vi "Servo Log change.vi"(10 "Servo variables Now":T3, 11 "Servo variables Before":T3) -> (2 "Changes":T1[](array[typedef]), 3 "Any change?":bool)   [LabVIEW 2017, in "Servo drive module.lvlib"]
doc: "Compares previous and current status variables of servo drives. Changes are concated into and array.\nparams:\nServo variables before\nServo variables now\nreturs:\nChanges"
uses:
  Servo drive module.lvlib
  ctl/Servo variables.ctl
  ctl/Status variable change.ctl
  ctl/Axis names.ctl
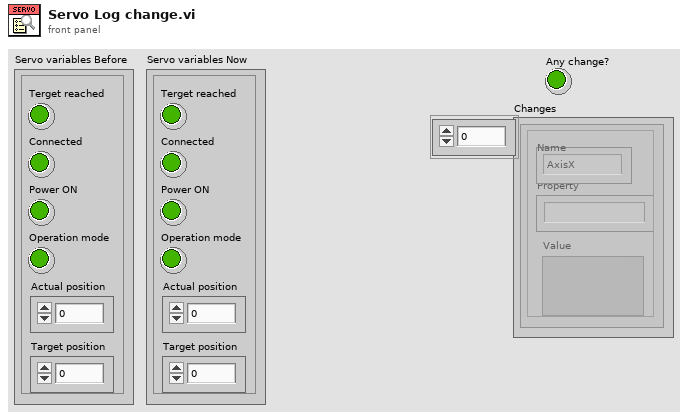
[diagram p1: front panel]
types:
  T1 = typedef "Servo drive module.lvlib/Status variable change.ctl" = cluster{"Property":string, "Value":variant, "Name":T2}
  T2 = typedef "Servo drive module.lvlib/Axis names.ctl" = enum16{"Unknown", "AxisX", "AxisY", "AxisZ_left", "AxisZ_middle", "AxisZ_right"}
  T3 = typedef "Servo drive module.lvlib/Servo variables.ctl" = cluster{"Terget reached":bool, "Connected":bool, "Power ON":bool, "Operation mode":bool, "Actual position":dbl, "Target position":dbl}
  T4 = cluster{"Terget reached":bool, "Connected":bool, "Power ON":bool, "Operation mode":bool, "Actual position":bool, "Target position":bool}
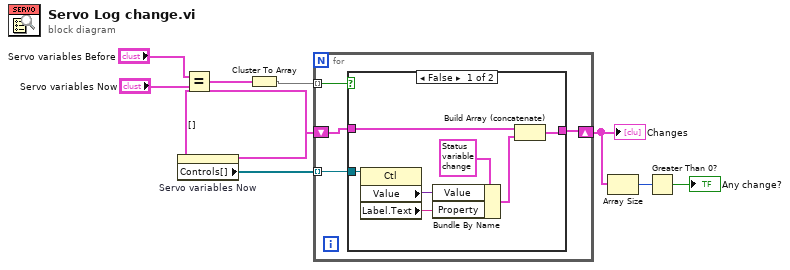
[diagram p0: block diagram]
diagram:
  n1 = property on="Servo variables Now" class="Clust (strict)"() -> ("Controls[]"=w5:refnum<vi>[])  [unwired: 2 in, 2 out]
  n2 = Equal?(x="Servo variables Before", y="Servo variables Now") -> (x = y?=w7:T4)
  n3 = Cluster To Array(cluster=w7) -> (array=w6:bool[])
  n4 = for {
    tunnel: w6 -> [w13] mode=indexing
    tunnel: w5 -> [w12] mode=indexing
    shift-right: [w10] -> w1
    shift-left: T1[] [] ("Array") -> [w11]
    n5 = case shown="False" w13 {
      tunnel: w12 -> [w20 _]
      tunnel: w11 -> [w18 w21]
      tunnel: [w17 w21] -> w10
      frame False {
        n6 = property class="Ctl"(reference=w20) -> ("Value"=w15:variant, "Label.Text"=w14:string)  [unwired: 1 in, 2 out]
        n7 = Bundle By Name(cluster=T1 {"Property"="", "Value"=variant, "Name"=enum."AxisX"} ("Array"), "Value"=w15, "Property"=w14) -> (w16:T1)
        n8 = Build Array (concatenate)(w18, w16) -> (w17:T1[])
      }
      frame True {
      }
    }
  }
  "Changes" <- w1
  n9 = Array Size(array=w1) -> (size(s)=w4:i32)
  n10 = Greater Than 0?(x=w4) -> (x > 0?=→"Any change?":bool)
